vi "Test TCRS Temperature Ramping Down.vi"(8 "error in (no error)":errorcluster, 11 "Thermal Chamber Response Simlator Test In":refnum<class "Thermal Chamber Response Simlator Test.lvclass">) -> (0 "error out":errorcluster, 3 "Thermal Chamber Response Simlator Test Out":refnum<class "Thermal Chamber Response Simlator Test.lvclass">)   [LabVIEW 2020, in "Thermal Chamber Response Simlator Test.lvclass"]
uses:
  Thermal Chamber Response Simlator Test.lvclass
  C:/Program Files (x86)/National Instruments/LabVIEW 2020/vi.lib/Asteme/LUnit/Test Case.lvclass
  Thermal Chamber Response Simlator/Thermal Chamber Response Simlator.lvclass
  Thermal Chamber Response Simlator/Thermal Chamber Response Simlator.lvclass/Thermal Chamber Response Simlator.ctl
  <vilib>/Asteme/LUnit/Test Case.lvclass/Test Case.ctl
  <vilib>/Asteme/LUnit/LUnit Assertion Result.lvclass/LUnit Assertion Result.ctl
  <vilib>/Asteme/LUnit/Palette/Pass.vi
  <vilib>/Asteme/LUnit/Palette/Fail.vi
  <vilib>/Asteme/LUnit/Variant to string.vi
  <vilib>/Asteme/LUnit/Set Assertion Type.vi
  <vilib>/Asteme/LUnit/Add test result.vi
  <vilib>/Asteme/LUnit/LUnit Write Passed.vi
  <vilib>/Asteme/LUnit/LUnit Get Test Case.vi
  <vilib>/Asteme/LUnit/Assertion Result/LUnit Get Test Name.vi
  <vilib>/Asteme/LUnit/LUnit Write Message.vi
  <vilib>/Asteme/LUnit/LUnit Write Description.vi
  <vilib>/Asteme/LUnit/LUnit Write Assertion Type.vi
  <vilib>/Asteme/LUnit/Read Test Case Name.vi
  Thermal Chamber Response Simlator/Private/Get Current Time if Not Set.vi
  <vilib>/Utility/Data Type/Get Type Information.vi
  <vilib>/Utility/LVClass/Get LV Class Name.vi
  <vilib>/Asteme/LUnit/LUnit Assertion Result.lvclass
  <vilib>/Asteme/LUnit/Test Case.lvclass
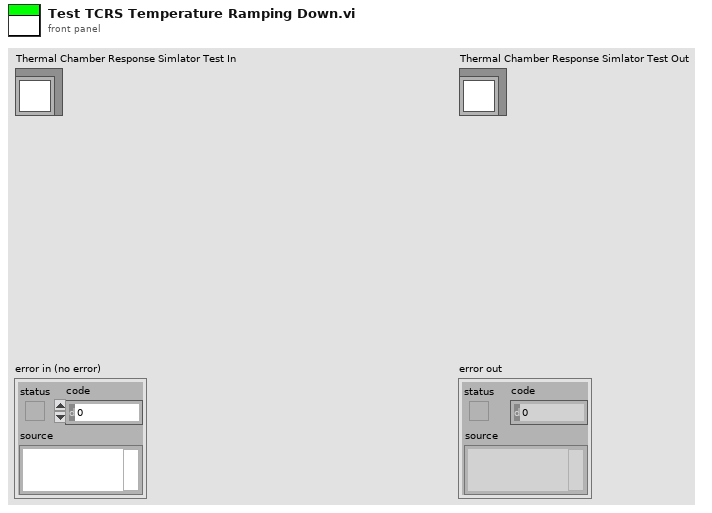
[diagram p1: front panel]
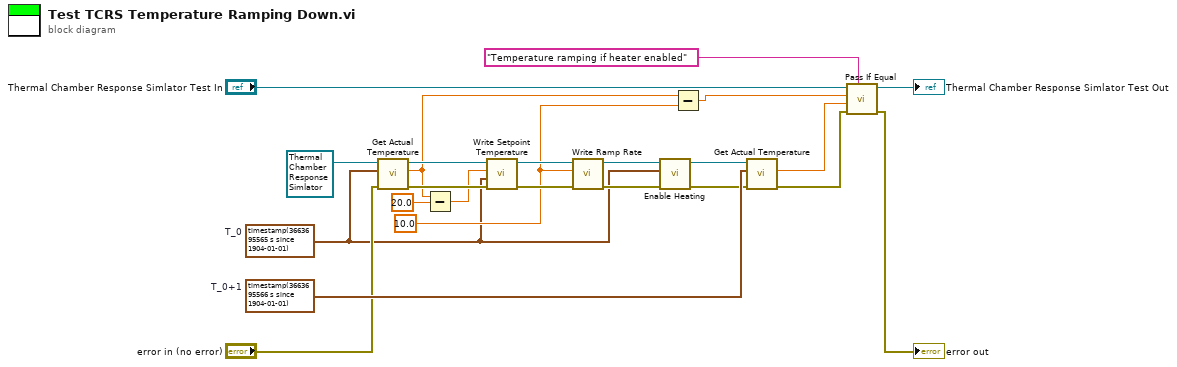
[diagram p0: block diagram]
diagram:
  w19 = timestamp(3663695566 s since 1904-01-01)  # T_0+1
  w4 = 10.0 ("Ramp Rate [degC/s]")
  w1 = timestamp(3663695565 s since 1904-01-01)  # T_0
  n1 = call "Get Actual Temperature.vi"("error in (no error)"="error in (no error)", "Time Stamp"=w1, "Thermal Chamber Response Simlator In"=refnum<class "Thermal Chamber Response Simlator.lvclass"> refnum ("Thermal Chamber Response Simlator.lvclass")) -> ("error out"=w21:errorcluster, "Actual Temperature [degC]"=w5:dbl, "Thermal Chamber Response Simlator Out"=w7:refnum<class "Thermal Chamber Response Simlator.lvclass">)  [unwired: 6 in]
  n2 = Subtract(x=w5, y=20.0) -> (x-y=w3:dbl)
  n3 = call "Write Setpoint Temperature.vi"("error in (no error)"=w21, "Update Time"=w1, "Setpoint Temperature [degC]"=w3, "Thermal Chamber Response Simlator In"=w7) -> ("error out"=w8:errorcluster, "Thermal Chamber Response Simlator Out"=w6:refnum<class "Thermal Chamber Response Simlator.lvclass">)  [unwired: 6 in]
  n4 = call "Write Ramp Rate.vi"("error in (no error)"=w8, "Ramp Rate [degC/s]"=w4, "Thermal Chamber Response Simlator In"=w6) -> ("error out"=w20:errorcluster, "Thermal Chamber Response Simlator Out"=w11:refnum<class "Thermal Chamber Response Simlator.lvclass">)  [unwired: 7 in]
  n5 = call "Enable Heating.vi"("error in (no error)"=w20, "Start Time"=w1, "Thermal Chamber Response Simlator In"=w11) -> ("error out"=w12:errorcluster, "Thermal Chamber Response Simlator Out"=w10:refnum<class "Thermal Chamber Response Simlator.lvclass">)  [unwired: 7 in]
  n6 = Subtract(x=w5, y=w4) -> (x-y=w9:dbl)
  n7 = call "Get Actual Temperature.vi"("error in (no error)"=w12, "Time Stamp"=w19, "Thermal Chamber Response Simlator In"=w10) -> ("error out"=w17:errorcluster, "Actual Temperature [degC]"=w16:dbl)  [unwired: 6 in, 1 out]
  n8 = call <vilib>:"Pass If Equal.vi"("Description"="Temperature ramping if heater enabled", "error in (no error)"=w17, "Actual"=w16, "Expected"=w9, "Test Case In"="Thermal Chamber Response Simlator Test In") -> ("error out"=→"error out":errorcluster, "Test Case Out"=→"Thermal Chamber Response Simlator Test Out":refnum<class "Thermal Chamber Response Simlator Test.lvclass">)  [unwired: 5 in]
